vi "DataTimeStr (SubVI).vi"() -> (3 "DataTimeStr":string)   [LabVIEW 2017]
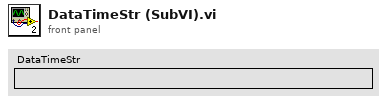
[diagram p1: front panel]
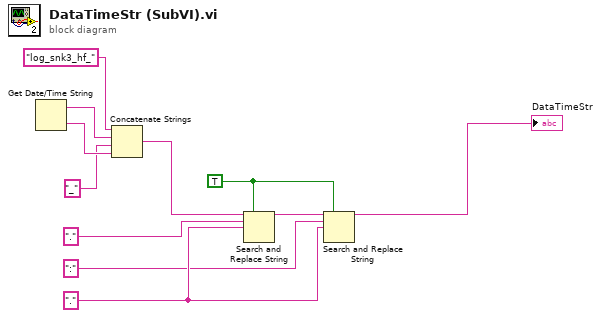
[diagram p0: block diagram]
diagram:
  w4 = TRUE ("replace all? (F)")
  w3 = "." ("replace string (\"\")")
  n1 = Get Date/Time String() -> (date string=w11:string, time string=w10:string)  [unwired: 3 in]
  n2 = Concatenate Strings("log_snk3_hf_" ("string"), w11, "_" ("string"), w10) -> (w8:string)
  n3 = Search and Replace String(replace all?=w4, input string=w8, search string=".", replace string=w3) -> (result string=w6:string)  [unwired: 4 in, 3 out]
  n4 = Search and Replace String(replace all?=w4, input string=w6, search string=":", replace string=w3) -> (result string=→"DataTimeStr":string)  [unwired: 4 in, 3 out]
